vi "SIM_Drive_MODULE_INIT.vi"(3 "Module Index":i32, 4 "SwerveRadiansPerCount":dbl=1.0, 5 "Drive PWM Channel":T2, 6 "DriveDistPerCount":dbl=1.0, 7 "Swerve PWM Channel":T2, 8 "Swerve B Channel":T1, 9 "Swerver A Channel":T1, 10 "Drive B Channel":T1, 11 "Drive A channel":T1) -> ()   [LabVIEW 2023]
uses:
  SIM_Drive_Globals.vi
  <vilib>/Rock Robotics/SystemInterfaces/DIO/FPGA_DIOChannel.ctl
  <vilib>/Rock Robotics/SystemInterfaces/DIO/FPGA_DIOPWMChannel.ctl
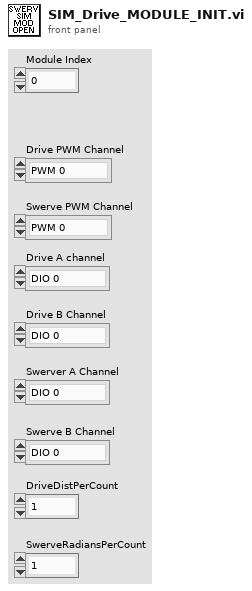
[diagram p1: front panel]
types:
  T1 = typedef "FPGA_DIOChannel.ctl" = enum8{"DIO 0", "DIO 1", "DIO 2", "DIO 3", "DIO 4", "DIO 5", "DIO 6", "DIO 7", "DIO 8", "DIO 9", "DIO MXP 0", "DIO MXP 1", "DIO MXP 2", "DIO MXP 3", "DIO MXP 4", "DIO MXP 5", "DIO MXP 6", "DIO MXP 7", "DIO MXP 8", "DIO MXP 9", "DIO MXP 10", "DIO MXP 11", "DIO MXP 12", "DIO MXP 13", "DIO MXP 14", "DIO MXP 15", "SPI Port CS1", "SPI Port CS2", "SPI Port CS3", "SPI Port MISO", "SPI Port MOSI", "Invalid"}
  T2 = typedef "FPGA_DIOPWMChannel.ctl" = enum8{"PWM 0", "PWM 1", "PWM 2", "PWM 3", "PWM 4", "PWM 5", "PWM 6", "PWM 7", "PWM 8", "PWM 9", "PWM MXP 0", "PWM MXP 1", "PWM MXP 2", "PWM MXP 3", "PWM MXP 4", "PWM MXP 5", "PWM MXP 6", "PWM MXP 7", "PWM MXP 8", "PWM MXP 9", "Invalid"}
  T3 = cluster{"Swerve Motor Device Index":i32, "Drive Motor Device Index":i32, "Swerve Encoder Device Index":i32, "Drive Encoder Device Index":i32, "Drive DistPerzcount":dbl, "SwerveRadPerCount":dbl}[]
  T4 = cluster{"Swerve Motor Device Index":i32, "Drive Motor Device Index":i32, "Swerve Encoder Device Index":i32, "Drive Encoder Device Index":i32, "Drive DistPerzcount":dbl, "SwerveRadPerCount":dbl}
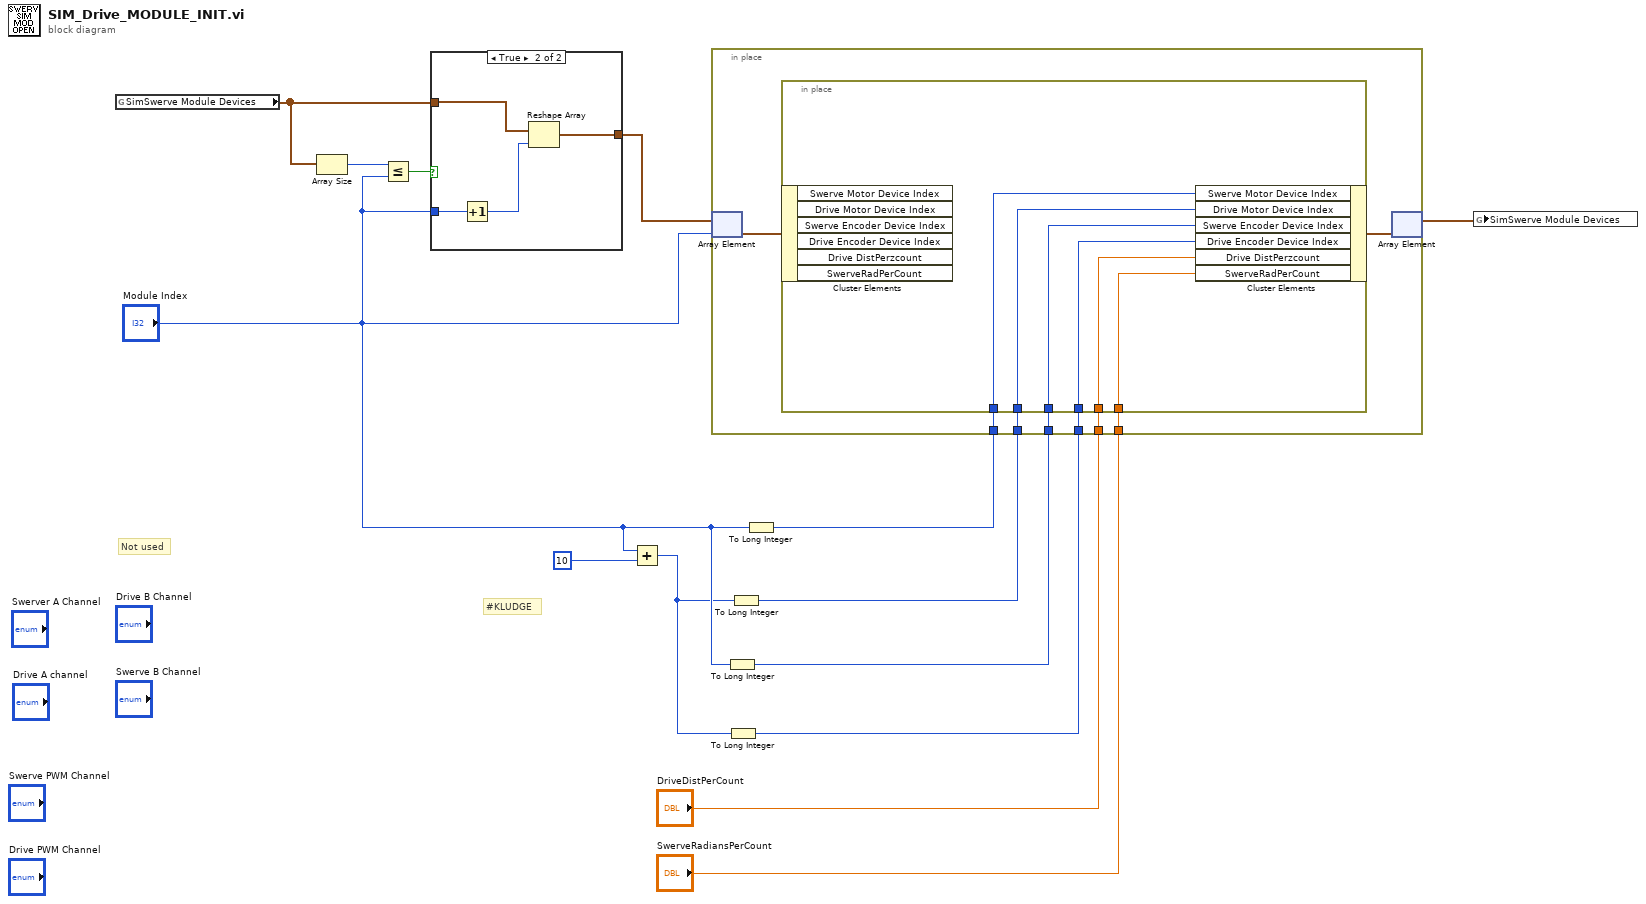
[diagram p0: block diagram]
diagram:
  # "#KLUDGE"
  # "Not used"
  n1 = global read "SIM_Drive_Globals.vi" "SimSwerve Module Devices"() -> (w5:T3)
  n2 = Array Size(array=w5) -> (size(s)=w7:i32)
  n3 = Less Or Equal?(x=w7, y="Module Index") -> (x <= y?=w6:bool)
  n4 = case shown="True" w6 {
    tunnel: w5 -> [w15 w17]
    tunnel: "Module Index" -> [_ w19]
    tunnel: [w15 w16] -> w4
    frame False {
    }
    frame True {
      n5 = Increment(x=w19) -> (x+1=w18:i32)
      n6 = Reshape Array(w17, w18) -> (w16:T3)
    }
  }
  n7 = Add(x="Module Index", y=10) -> (x+y=w1:i32)
  n8 = To Long Integer(number="Module Index") -> (32bit integer=w11:i32)
  n9 = To Long Integer(number=w1) -> (32bit integer=w10:i32)
  n10 = To Long Integer(number=w1) -> (32bit integer=w12:i32)
  n11 = To Long Integer(number="Module Index") -> (32bit integer=w13:i32)
  n12 = in-place {
    in-place-border: w13 -> [w26]
    in-place-border: w12 -> [w25]
    in-place-border: w11 -> [w23]
    in-place-border: w10 -> [w22]
    in-place-border: "DriveDistPerCount" -> [w21]
    in-place-border: "SwerveRadiansPerCount" -> [w20]
    n13 = in-place-array #1(w4, "Module Index") -> (w27:T4)
    n14 = in-place {
      in-place-border: w26 -> [w33]
      in-place-border: w25 -> [w32]
      in-place-border: w23 -> [w31]
      in-place-border: w22 -> [w30]
      in-place-border: w21 -> [w29]
      in-place-border: w20 -> [w28]
      n15 = in-place-cluster #2(w27) -> ()  [unwired: 6 out]
      n16 = in-place-cluster #2("Swerve Motor Device Index"=w33, "Drive Motor Device Index"=w32, "Swerve Encoder Device Index"=w31, "Drive Encoder Device Index"=w30, "Drive DistPerzcount"=w29, "SwerveRadPerCount"=w28) -> (w24:T4)
    }
    n17 = in-place-array #1(w24) -> (w14:T3)  [unwired: 1 out]
  }
  n18 = global write "SIM_Drive_Globals.vi" "SimSwerve Module Devices"(w14) -> ()
